vi "Initialize Instrument.vi"(8 "error in (no error)":errorcluster, 10 "Reset":bool, 11 "Keithley 24xx in":refnum<class "Keithley 24xx.lvclass">) -> (0 "error out":errorcluster, 3 "Keithley 24xx out":refnum<class "Keithley 24xx.lvclass">)   [LabVIEW 2020, in "Keithley 24xx.lvclass"]
uses:
  Keithley 24xx.lvclass
  C:/Sandbox/Git_Sandbox/WiSpry Test Framework source code (LV20)/WiSpry Test Framework/Instruments/Instrument.lvclass
  C:/Sandbox/Git_Sandbox/WiSpry Test Framework source code (LV20)/WiSpry Test Framework/Instruments/Power Supply/Power Supply.lvclass
  Instrument.lvclass/Instrument.ctl
  Power Supply.lvclass/Power Supply.ctl
  Instrument.lvclass
  <instrlib>/Keithley 24XX/Keithley 24XX.lvlib
  Power Supply.lvclass
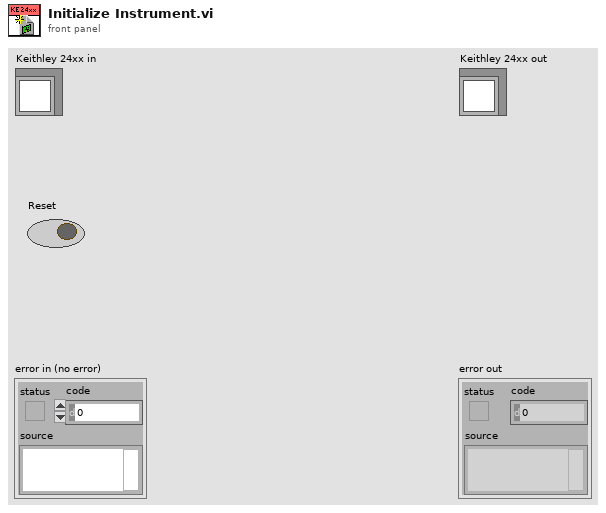
[diagram p1: front panel]
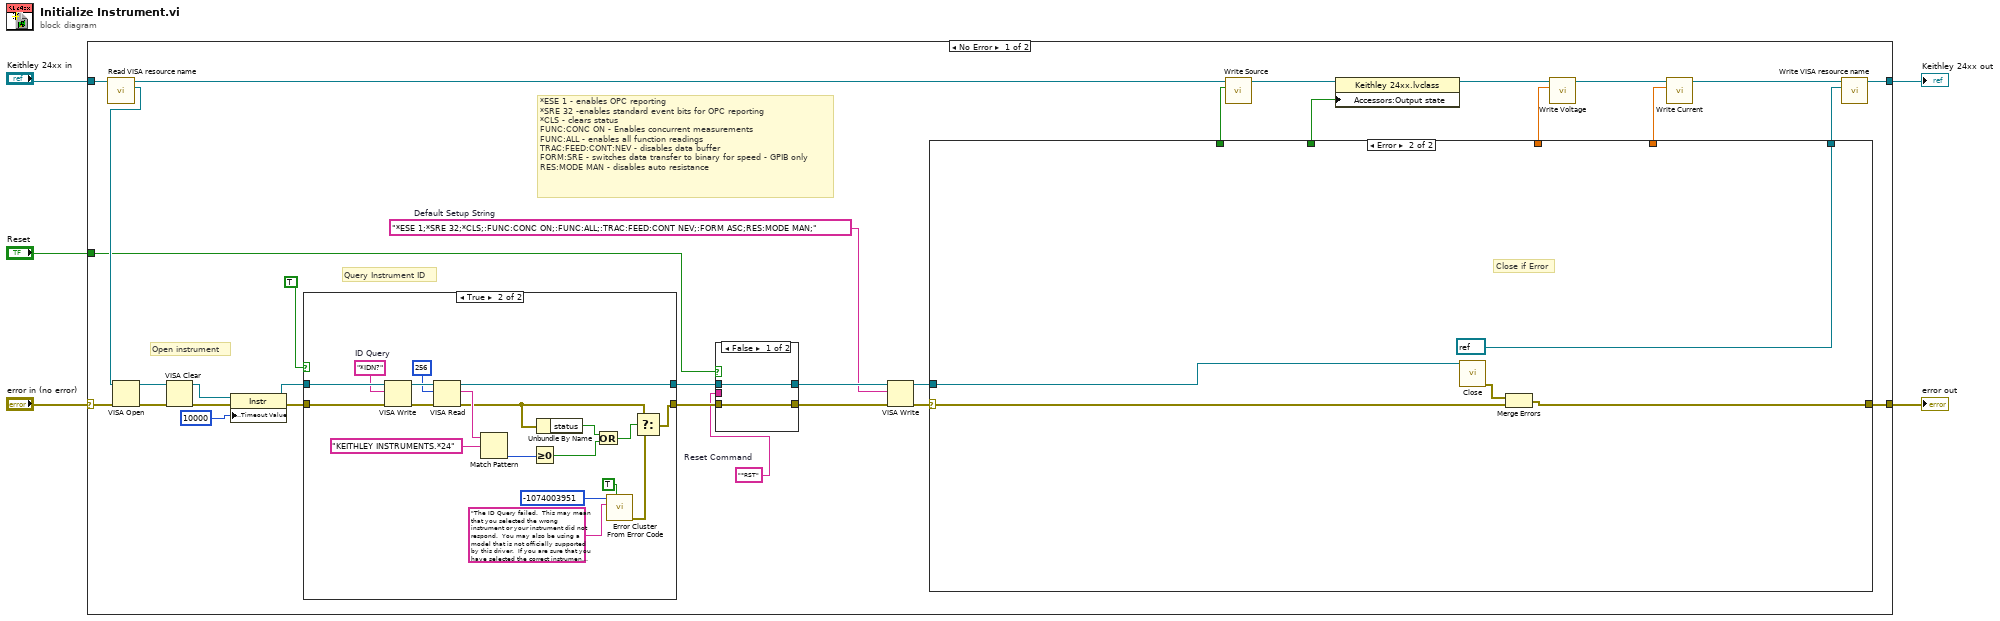
[diagram p0: block diagram]
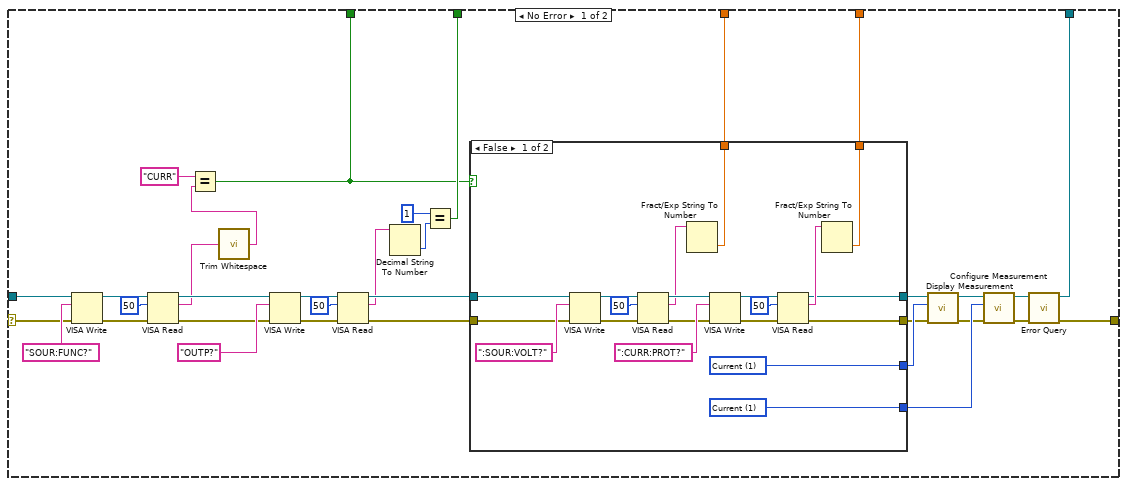
[diagram p2: hidden frame]
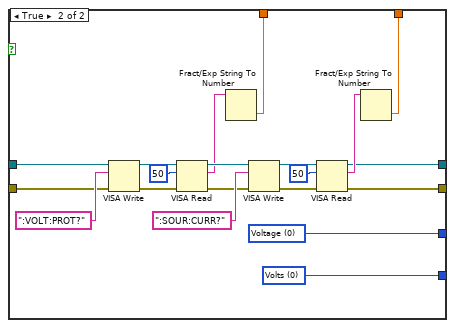
[diagram p3: hidden frame]
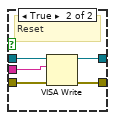
[diagram p4: hidden frame]
diagram:
  n1 = case shown="No Error" "error in (no error)" {
    selector: "error in (no error)" -> [w15 w146]
    tunnel: [w36 w146] -> w3
    tunnel: [w37 w145] -> w4
    tunnel: "Reset" -> [w7 _]
    tunnel: "Keithley 24xx in" -> [w34 w145]
    frame No Error {
      w8 = "*ESE 1;*SRE 32;*CLS;:FUNC:CONC ON;:FUNC:ALL;:TRAC:FEED:CONT NEV;:FORM ASC;RES:MODE MAN;"  # Default Setup String
      w13 = "*RST"  # Reset Command
      # "*ESE 1 - enables OPC reporting\n*SRE 32 -enables standard event bits for OPC reporting\n*CLS - clears status\nFUNC:CONC ON - Enables concurrent measurements\nFUNC:ALL - enables all function readings\nTRAC:FEED:CONT:NEV - disables data buffer\nFORM:SRE - switches data transfer to binary for speed - GPIB only\nRES:MODE MAN - disables auto resistance"
      # "Query Instrument ID"
      # "Open instrument"
      n2 = call "Read VISA resource name.vi"("Instrument in"=w34) -> ("VISA resource name"=w14:refnum<visa-resource-name>, "Instrument out"=w28:refnum<class "Keithley 24xx.lvclass">)  [unwired: 9 in]
      n3 = VISA Open(error in (no error)=w15, VISA resource name=w14) -> (VISA resource name=w19:refnum<visa-resource-name>, error out=w18:errorcluster)  [unwired: 3 in]
      n4 = VISA Clear(VISA resource name=w19, error in (no error)=w18) -> (VISA resource name out=w17:refnum<visa-resource-name>, error out=w16:errorcluster)
      n5 = property class="Instr"(reference=w17, error in=w16, "General Settings:Timeout Value"=u32 10000) -> (reference out=w21:refnum<visa-resource-name>, error out=w20:errorcluster)
      n6 = case shown="True" TRUE ("ID Query (True)") {
        tunnel: [w124 w144] -> w24
        tunnel: [w125 w141] -> w25
        tunnel: w21 -> [w125 w142]
        tunnel: w20 -> [w124 w143]
        frame False {
        }
        frame True {
          w135 = "*IDN?"  # ID Query
          n7 = VISA Write(VISA resource name=w142, write buffer=w135, error in (no error)=w143) -> (VISA resource name out=w139:refnum<visa-resource-name>, error out=w138:errorcluster)  [unwired: 1 out]
          n8 = VISA Read(VISA resource name=w139, byte count=u32 256, error in (no error)=w138) -> (VISA resource name out=w141:refnum<visa-resource-name>, read buffer=w140:string, error out=w129:errorcluster)  [unwired: 1 out]
          n9 = Match Pattern(string=w140, regular expression="KEITHLEY INSTRUMENTS.*24") -> (offset past match=w130:i32)  [unwired: 1 in, 3 out]
          n10 = Greater Or Equal To 0?(x=w130) -> (x >= 0?=w127:bool)
          n11 = Unbundle By Name(w129) -> ("status"=w128:bool)
          n12 = Or(x=w128, y=w127) -> (x .or. y?=w126:bool)
          n13 = call <vilib>:"Error Cluster From Error Code.vi"("show call chain? (False)"=TRUE, "error message (\"\")"="The ID Query failed.  This may mean that you selected the wrong instrument or your instrument did not respond.  You may also be using a model that is not officially supported by this driver.  If you are sure that you have selected the correct instrument and it is responding, try disabling the ID Query." ("Source (VI Name)"), "error code (0)"=-1074003951 ("Code")) -> ("error out"=w134:errorcluster)  [unwired: 6 in]
          n14 = Select(t=w129, s=w126, f=w134) -> (s? t:f=w144:errorcluster)
        }
      }
      n15 = case shown="False" w7 {
        tunnel: w24 -> [w117 w122]
        tunnel: [w117 w119] -> w12
        tunnel: w25 -> [w118 w121]
        tunnel: [w118 w120] -> w11
        tunnel: w13 -> [_ w123]
        frame False {
        }
        frame True {
          # "Reset"
          n16 = VISA Write(VISA resource name=w121, write buffer=w123, error in (no error)=w122) -> (VISA resource name out=w120:refnum<visa-resource-name>, error out=w119:errorcluster)  [unwired: 1 out]
        }
      }
      n17 = VISA Write(VISA resource name=w11, write buffer=w8, error in (no error)=w12) -> (VISA resource name out=w9:refnum<visa-resource-name>, error out=w10:errorcluster)  [unwired: 1 out]
      n18 = case shown="Error" w10 {
        selector: w10 -> [w42 w113]
        tunnel: [w39 w112] -> w36
        tunnel: [w38 refnum<visa-resource-name> refnum ("VISA resource name out")] -> w35
        tunnel: [w49 _] -> w31
        tunnel: [w48 _] -> w30
        tunnel: [w47 _] -> w6
        tunnel: [w46 _] -> w26
        tunnel: w9 -> [w43 w116]
        frame No Error {
          n19 = VISA Write(VISA resource name=w43, write buffer="SOUR:FUNC?", error in (no error)=w42) -> (VISA resource name out=w56:refnum<visa-resource-name>, error out=w55:errorcluster)  [unwired: 1 out]
          n20 = VISA Read(VISA resource name=w56, byte count=u32 50, error in (no error)=w55) -> (VISA resource name out=w53:refnum<visa-resource-name>, read buffer=w45:string, error out=w54:errorcluster)  [unwired: 1 out]
          n21 = call <vilib>:"Trim Whitespace.vi"("string"=w45) -> ("trimmed string"=w44:string)  [unwired: 1 in]
          n22 = Equal?(x="CURR", y=w44) -> (x = y?=w46:bool)
          n23 = VISA Write(VISA resource name=w53, write buffer="OUTP?", error in (no error)=w54) -> (VISA resource name out=w67:refnum<visa-resource-name>, error out=w66:errorcluster)  [unwired: 1 out]
          n24 = VISA Read(VISA resource name=w67, byte count=u32 50, error in (no error)=w66) -> (VISA resource name out=w63:refnum<visa-resource-name>, read buffer=w61:string, error out=w62:errorcluster)  [unwired: 1 out]
          n25 = Decimal String To Number(string=w61) -> (number=w60:i32)  [unwired: 2 in, 1 out]
          n26 = Equal?(x=1, y=w60) -> (x = y?=w47:bool)
          n27 = case shown="False" w46 {
            tunnel: [w91 w111] -> w71
            tunnel: [w90 w110] -> w68
            tunnel: w63 -> [w81 w101]
            tunnel: w62 -> [w80 w100]
            tunnel: [w75 w95] -> w52
            tunnel: [w74 w94] -> w51
            tunnel: [w73 w93] -> w49
            tunnel: [w72 w92] -> w48
            frame False {
              w90 = u16 1 items=["Voltage", "Current", "Resistance"] ("Displayed Measurement (0: Voltage)")
              w91 = u16 1 items=["Volts", "Current", "Resistance"] ("Function (0: Volts)")
              n28 = VISA Write(VISA resource name=w81, write buffer=":SOUR:VOLT?", error in (no error)=w80) -> (VISA resource name out=w86:refnum<visa-resource-name>, error out=w87:errorcluster)  [unwired: 1 out]
              n29 = VISA Read(VISA resource name=w86, byte count=u32 50, error in (no error)=w87) -> (VISA resource name out=w79:refnum<visa-resource-name>, read buffer=w76:string, error out=w78:errorcluster)  [unwired: 1 out]
              n30 = Fract/Exp String To Number(string=w76) -> (number=w73:dbl)  [unwired: 3 in, 1 out]
              n31 = VISA Write(VISA resource name=w79, write buffer=":CURR:PROT?", error in (no error)=w78) -> (VISA resource name out=w85:refnum<visa-resource-name>, error out=w84:errorcluster)  [unwired: 1 out]
              n32 = VISA Read(VISA resource name=w85, byte count=u32 50, error in (no error)=w84) -> (VISA resource name out=w74:refnum<visa-resource-name>, read buffer=w77:string, error out=w75:errorcluster)  [unwired: 1 out]
              n33 = Fract/Exp String To Number(string=w77) -> (number=w72:dbl)  [unwired: 3 in, 1 out]
            }
            frame True {
              w110 = u16 0 items=["Voltage", "Current", "Resistance"] ("Displayed Measurement (0: Voltage)")
              w111 = u16 0 items=["Volts", "Current", "Resistance"] ("Function (0: Volts)")
              n34 = VISA Write(VISA resource name=w101, write buffer=":VOLT:PROT?", error in (no error)=w100) -> (VISA resource name out=w106:refnum<visa-resource-name>, error out=w107:errorcluster)  [unwired: 1 out]
              n35 = VISA Read(VISA resource name=w106, byte count=u32 50, error in (no error)=w107) -> (VISA resource name out=w99:refnum<visa-resource-name>, read buffer=w96:string, error out=w98:errorcluster)  [unwired: 1 out]
              n36 = Fract/Exp String To Number(string=w96) -> (number=w93:dbl)  [unwired: 3 in, 1 out]
              n37 = VISA Write(VISA resource name=w99, write buffer=":SOUR:CURR?", error in (no error)=w98) -> (VISA resource name out=w105:refnum<visa-resource-name>, error out=w104:errorcluster)  [unwired: 1 out]
              n38 = VISA Read(VISA resource name=w105, byte count=u32 50, error in (no error)=w104) -> (VISA resource name out=w94:refnum<visa-resource-name>, read buffer=w97:string, error out=w95:errorcluster)  [unwired: 1 out]
              n39 = Fract/Exp String To Number(string=w97) -> (number=w92:dbl)  [unwired: 3 in, 1 out]
            }
          }
          n40 = call <instrlib>:"Display Measurement.vi"("error in (no error)"=w52, "Displayed Measurement (0: Voltage)"=w68, "VISA resource name"=w51) -> ("error out"=w69:errorcluster, "VISA resource name out"=w70:refnum<visa-resource-name>)  [unwired: 7 in]
          n41 = call <instrlib>:"Configure Measurement.vi"("error in (no error)"=w69, "Function (0: Volts)"=w71, "VISA resource name"=w70) -> ("error out"=w40:errorcluster, "VISA resource name out"=w41:refnum<visa-resource-name>)  [unwired: 7 in]
          n42 = call <instrlib>:"Error Query.vi"("error in (no error)"=w40, "VISA resource name"=w41) -> ("error out"=w39:errorcluster, "VISA resource name out"=w38:refnum<visa-resource-name>)  [unwired: 6 in, 2 out]
        }
        frame Error {
          # "Close if Error"
          n43 = call <instrlib>:"Close.vi"("VISA resource name"=w116) -> ("error out"=w114:errorcluster)  [unwired: 10 in]
          n44 = Merge Errors(w114, w113) -> (w112:errorcluster)
        }
      }
      n45 = call-dynamic "Write Source.vi"("Source"=w26, "Power Supply in"=w28) -> ("Power Supply out"=w29:refnum<class "Keithley 24xx.lvclass">)  [unwired: 9 in]
      n46 = property class="Keithley 24xx.lvclass"(reference=w29, "Accessors:Output state"=w6) -> (reference out=w33:refnum<class "Keithley 24xx.lvclass">)  [unwired: 1 in, 1 out]
      n47 = call "Write Voltage.vi"("Voltage"=w31, "Power Supply in"=w33) -> ("Power Supply out"=w32:refnum<class "Keithley 24xx.lvclass">)  [unwired: 9 in]
      n48 = call "Write Current.vi"("Current"=w30, "Power Supply in"=w32) -> ("Power Supply out"=w27:refnum<class "Keithley 24xx.lvclass">)  [unwired: 9 in]
      n49 = call "Write VISA resource name.vi"("VISA resource name"=w35, "Instrument in"=w27) -> ("Instrument out"=w37:refnum<class "Keithley 24xx.lvclass">)  [unwired: 9 in]
    }
    frame Error {
    }
  }
  "error out" <- w3
  "Keithley 24xx out" <- w4
